vi "密码比对程序.vi"(6 "密码":string="456\n", 7 "账户":string="123", 8 "原密码所在位置":path=path "E:/桌面/Desktop/登录测试/user.txt") -> (2 "x = y?":bool)   [LabVIEW 2015]
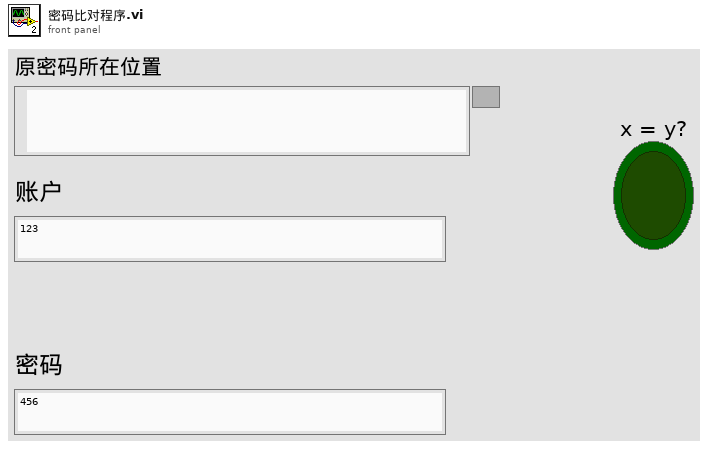
[diagram p1: front panel]
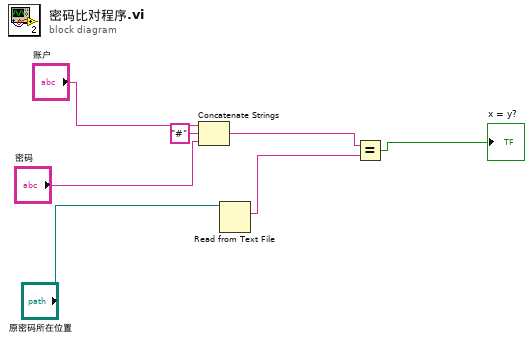
[diagram p0: block diagram]
diagram:
  n1 = Concatenate Strings("账户", "#" ("字符串"), "密码") -> (w6:string)
  n2 = Read from Text File(file (use dialog)="原密码所在位置") -> (text=w5:string)  [unwired: 3 in, 3 out]
  n3 = Equal?(x=w6, y=w5) -> (x = y?=→"x = y?":bool)
